vi "Turn to Angle.vi"(6 "in power":dbl, 8 "error in (no error)":errorcluster, 10 "Angle":dbl, 11 "RobotDriveDevRef":T1={"DevStatus"={"status"=FALSE, "code"=0, "source"=""}, "Motors[]"=[], "Square Inputs"=FALSE, "Max Output"=1.0}) -> (0 "error out":errorcluster, 1 "out power":dbl, 3 "ref Num":T1={"DevStatus"={"status"=FALSE, "code"=0, "source"=""}, "Motors[]"=[], "Square Inputs"=FALSE, "Max Output"=1.0})   [LabVIEW 2017]
uses:
  <vilib>/Rock Robotics/WPI/RobotDrive/WPI_RobotDriveDevRef.ctl
  <vilib>/Rock Robotics/WPI/MotorControl/WPI_MotorControlDeviceRef.ctl
  <vilib>/Rock Robotics/WPI/MotorControl/WPI_MotorControlType.ctl
  <vilib>/Rock Robotics/SystemInterfaces/DIO/FPGA_DIOPWMChannel.ctl
  <vilib>/Rock Robotics/WPI/PWM/WPI_PWMDeadband.ctl
  <vilib>/Rock Robotics/SystemInterfaces/DIO/FPGA_DIOChannel.ctl
  Robot Global Data.vi
panel:
  out "difference":dbl
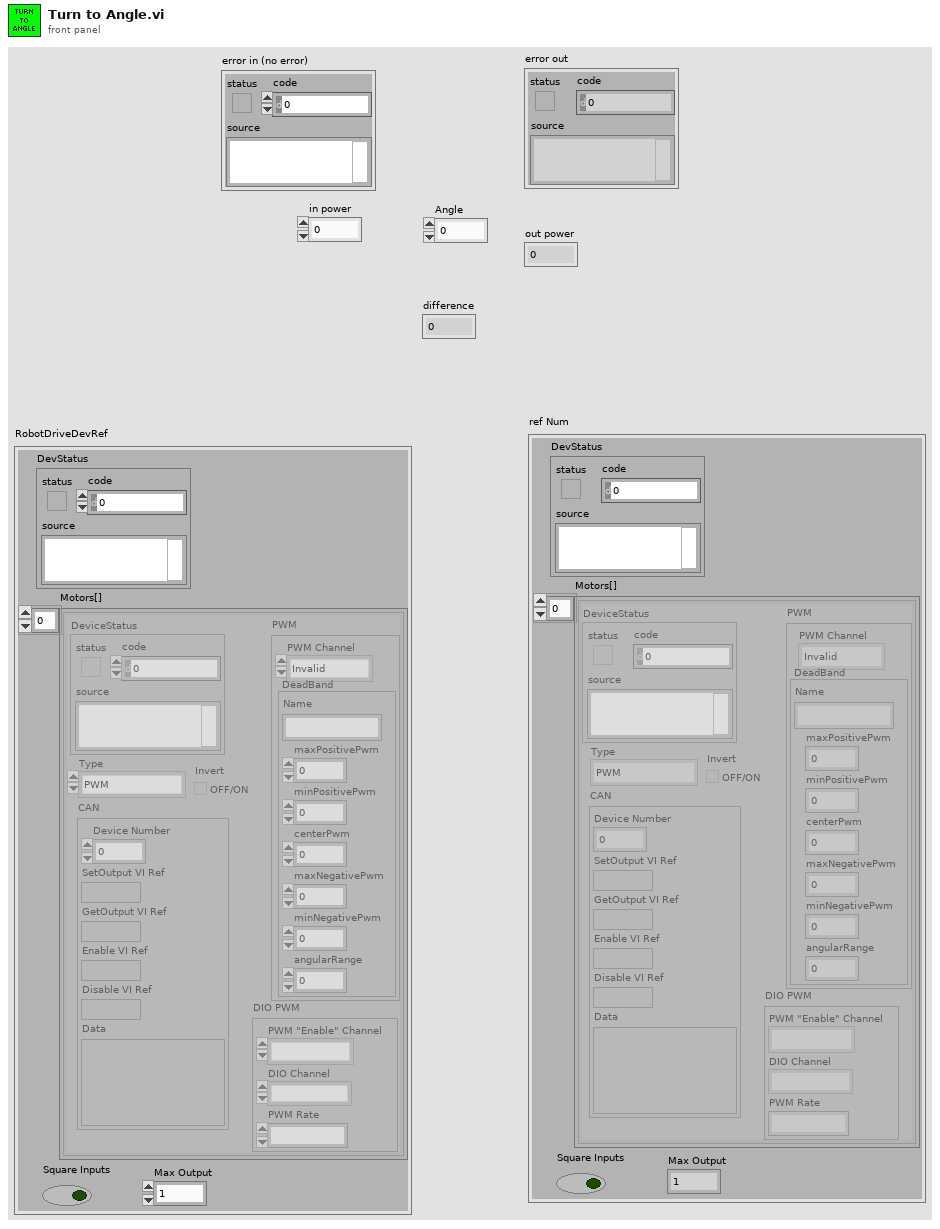
[diagram p1: front panel]
types:
  T1 = typedef "WPI_RobotDriveDevRef.ctl" = cluster{"DevStatus":errorcluster, "Motors[]":T2[], "Square Inputs":bool, "Max Output":dbl}
  T2 = typedef "WPI_MotorControlDeviceRef.ctl" = cluster{"DeviceStatus":errorcluster, "Type":T3, "PWM":cluster{"PWM Channel":T4, "DeadBand":T5}, "CAN":cluster{"Device Number":u8, "SetOutput VI Ref":variant, "GetOutput VI Ref":variant, "Enable VI Ref":variant, "Disable VI Ref":variant, "Data":variant}, "Invert":bool, "DIO PWM":cluster{"PWM \"Enable\" Channel":T4, "DIOChannel":T6, "PWM Rate":dbl}}
  T3 = typedef "WPI_MotorControlType.ctl" = enum16{"PWM", "CAN", "DIO PWM"}
  T4 = typedef "FPGA_DIOPWMChannel.ctl" = enum8{"PWM 0", "PWM 1", "PWM 2", "PWM 3", "PWM 4", "PWM 5", "PWM 6", "PWM 7", "PWM 8", "PWM 9", "PWM MXP 0", "PWM MXP 1", "PWM MXP 2", "PWM MXP 3", "PWM MXP 4", "PWM MXP 5", "PWM MXP 6", "PWM MXP 7", "PWM MXP 8", "PWM MXP 9", "Invalid"}
  T5 = typedef "WPI_PWMDeadband.ctl" = cluster{"Name":string, "maxPositivePwm":i32, "minPositivePwm":i32, "centerPwm":i32, "maxNegativePwm":i32, "minNegativePwm":i32, "angularRange":u16}
  T6 = typedef "FPGA_DIOChannel.ctl" = enum8{"DIO 0", "DIO 1", "DIO 2", "DIO 3", "DIO 4", "DIO 5", "DIO 6", "DIO 7", "DIO 8", "DIO 9", "DIO MXP 0", "DIO MXP 1", "DIO MXP 2", "DIO MXP 3", "DIO MXP 4", "DIO MXP 5", "DIO MXP 6", "DIO MXP 7", "DIO MXP 8", "DIO MXP 9", "DIO MXP 10", "DIO MXP 11", "DIO MXP 12", "DIO MXP 13", "DIO MXP 14", "DIO MXP 15", "SPI Port CS1", "SPI Port CS2", "SPI Port CS3", "SPI Port MISO", "SPI Port MOSI", "Invalid"}
  T7 = cluster{"Yaw":dbl, "Roll":dbl, "Pitch":dbl, "Heading":dbl, "Fused Heading":dbl}
  T8 = typedef "WPI_EncoderDevRef.ctl" = cluster{"DevStatus":errorcluster, "EncoderIndex":T9, "CounterIndex":T10, "DistancePerCount":dbl, "Decoding Type":T11}
  T9 = typedef "FPGA_EncoderIdx.ctl" = enum8{"Enc 0", "Enc 1", "Enc 2", "Enc 3", "Enc 4", "Enc 5", "Enc 6", "Enc 7", "Invalid"}
  T10 = typedef "FPGA_CounterCtrSystemIndex.ctl" = enum8{"Ctr 0", "Ctr 1", "Ctr 2", "Ctr 3", "Ctr 4", "Ctr 5", "Ctr 6", "Ctr 7", "Invalid"}
  T11 = typedef "WPI_EncoderType.ctl" = enum16{"1x", "2x", "4x"}
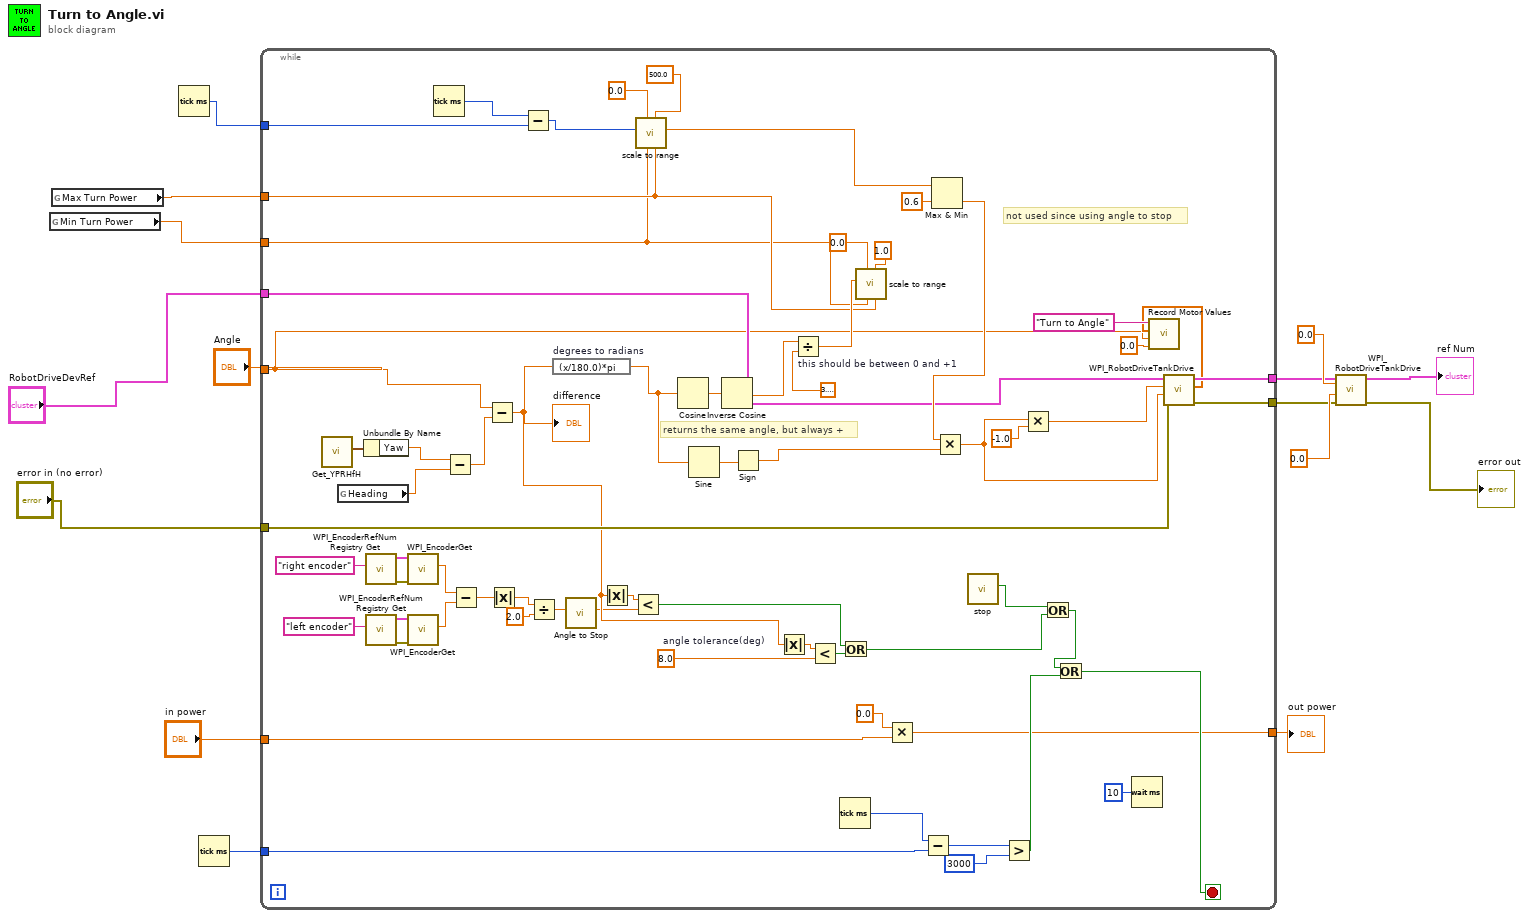
[diagram p0: block diagram]
diagram:
  n1 = global read "Robot Global Data.vi" "Min Turn Power"() -> (w5:dbl)
  n2 = global read "Robot Global Data.vi" "Max Turn Power"() -> (w6:dbl)
  n3 = Tick Count (ms)() -> (millisecond timer value=w9:u32)
  n4 = Tick Count (ms)() -> (millisecond timer value=w10:u32)
  n5 = while {
    tunnel: "Angle" -> [w40]
    tunnel: [w80] -> w12
    tunnel: [w79] -> w11
    tunnel: w10 -> [w73]
    tunnel: w9 -> [w58]
    tunnel: [w49] -> w7
    tunnel: "in power" -> [w50]
    tunnel: w6 -> [w47]
    tunnel: w5 -> [w46]
    tunnel: "RobotDriveDevRef" -> [w44]
    tunnel: "error in (no error)" -> [w43]
    stop <- w69 stop-if-true
    w77 = 8.0  # angle tolerance(deg)
    # "not used since using angle to stop"
    # "returns the same angle, but always +"
    n6 = call <vilib>:"Get_YPRHfH.vi"() -> ("YRPHfH"=w75:T7)  [unwired: 11 in]
    n7 = global read "Robot Global Data.vi" "Heading"() -> (w62:dbl)
    n8 = Unbundle By Name(w75) -> ("Yaw"=w63:dbl)
    n9 = call <vilib>:"WPI_EncoderRefNum Registry Get.vi"("refnum name"="right encoder") -> ("error out"=w38:errorcluster, "EncoderDevRef"=w37:T8)  [unwired: 9 in]
    n10 = call <vilib>:"WPI_EncoderRefNum Registry Get.vi"("refnum name"="left encoder") -> ("error out"=w35:errorcluster, "EncoderDevRef"=w34:T8)  [unwired: 9 in]
    n11 = call <vilib>:"WPI_EncoderGet.vi"("error in (no error)"=w38, "EncoderDevRef"=w37) -> ("Distance"=w25:dbl)  [unwired: 4 in, 5 out]
    n12 = call <vilib>:"WPI_EncoderGet.vi"("error in (no error)"=w35, "EncoderDevRef"=w34) -> ("Distance"=w24:dbl)  [unwired: 4 in, 5 out]
    n13 = Tick Count (ms)() -> (millisecond timer value=w60:u32)
    n14 = Subtract(x=w63, y=w62) -> (x-y=w61:dbl)
    n15 = Subtract(x=w25, y=w24) -> (x-y=w23:dbl)
    n16 = Subtract(x=w40, y=w61) -> (x-y=w31:dbl)
    "difference" <- w31
    n17 = Absolute Value(x=w23) -> (abs(x)=w22:dbl)
    n18 = Subtract(x=w60, y=w58) -> (x-y=w20:u32)
    n19 = Divide(x=w22, y=2.0) -> (x/y=w29:dbl)
    n20 = expression code="(x/180.0)*pi" "degrees to radians"(w31) -> (w65:dbl)
    n21 = call "Angle to Stop.vi"("Avg Speed"=w29) -> ("Angle"=w28:dbl)  [unwired: 10 in]
    n22 = Absolute Value(x=w31) -> (abs(x)=w30:dbl)
    n23 = Less?(x=w30, y=w28) -> (x < y?=w26:bool)
    n24 = call "scale to range.vi"("Max"=w47, "High"=500.0, "Min"=w46, "Low"=0.0, "In Signal"=w20) -> ("Output signal"=w19:dbl)  [unwired: 6 in]
    n25 = Cosine(x=w65) -> (cos(x)=w68:dbl)
    n26 = Sine(x=w65) -> (sin(x)=w67:dbl)
    n27 = Inverse Cosine(1:w68) -> (0:w56:dbl)
    n28 = Sign(1:w67) -> (0:w66:dbl)
    n29 = Absolute Value(x=w31) -> (abs(x)=w78:dbl)
    n30 = Divide "this should be between 0 and +1"(x=w56, y=3.141592653589793) -> (x/y=w53:dbl)
    n31 = Less?(x=w78, y=w77) -> (x < y?=w27:bool)
    n32 = Tick Count (ms)() -> (millisecond timer value=w74:u32)
    n33 = Or(x=w26, y=w27) -> (x .or. y?=w17:bool)
    n34 = call "scale to range.vi"("Max"=w47, "High"=1.0, "Min"=w46, "Low"=0.0, "In Signal"=w53) -> ()  [unwired: 6 in, 1 out]
    n35 = Multiply(x=0.0, y=w50) -> (x*y=w49:dbl)
    n36 = Subtract(x=w74, y=w73) -> (x-y=w72:u32)
    n37 = Max & Min(x=w19, y=0.6) -> (min(x,y)=w54:dbl)  [unwired: 1 out]
    n38 = Multiply(x=w54, y=w66) -> (x*y=w55:dbl)
    n39 = call "stop.vi"() -> ("Boolean"=w18:bool)  [unwired: 11 in]
    n40 = Greater?(x=w72, y=u32 3000) -> (0:w70:bool)
    n41 = Multiply(x=w55, y=-1.0) -> (x*y=w64:dbl)
    n42 = Or(x=w18, y=w17) -> (x .or. y?=w16:bool)
    n43 = Or(x=w16, y=w70) -> (x .or. y?=w69:bool)
    n44 = Wait (ms)(milliseconds to wait=u32 10) -> ()  [unwired: 1 out]
    n45 = call <vilib>:"WPI_RobotDriveTankDrive.vi"("error in (no error)"=w43, "Right axis value"=w55, "Left axis value"=w64, "RobotDriveDevRef"=w44) -> ("error out"=w79:errorcluster, "Motor Values"=w41:dbl[], "RobotDriveDevRef"=w80:T1)  [unwired: 5 in]
    n46 = call "Record Motor Values.vi"("Target1 2"=0.0, "Target1"=w40, "Motor Values"=w41, "VI Block Name"="Turn to Angle" ("string")) -> ()  [unwired: 8 in]
  }
  "out power" <- w7
  n47 = call <vilib>:"WPI_RobotDriveTankDrive.vi"("error in (no error)"=w11, "Right axis value"=0.0, "Left axis value"=0.0, "RobotDriveDevRef"=w12) -> ("error out"=→"error out":errorcluster, "RobotDriveDevRef"=→"ref Num":T1)  [unwired: 5 in, 1 out]
